vi "ReserveDbServer.vi"(0 "DashboardServer in":refnum<class "Dashboard Server.lvclass">, 5 "error in (no error)":errorcluster) -> (14 "DashboardServer out":refnum<class "Dashboard Server.lvclass">, 19 "error out":errorcluster)   [LabVIEW 2019, in "Dashboard Server.lvclass"]
uses:
  Dashboard Server.lvclass
  Dashboard Server.lvclass/Dashboard Server.ctl
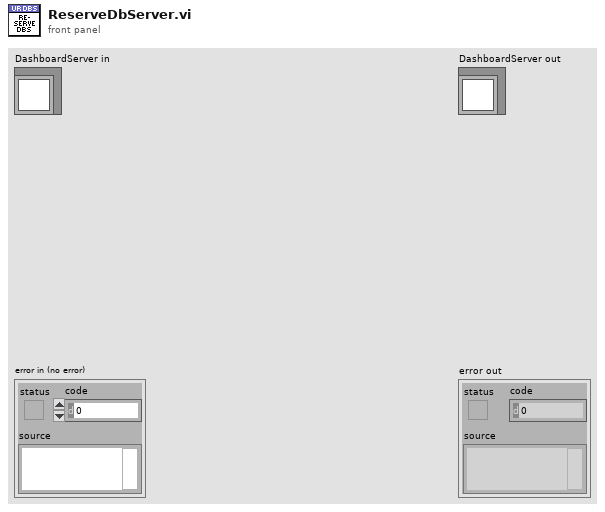
[diagram p1: front panel]
types:
  T1 = typedef "Semaphore RefNum" = refnum<k1>
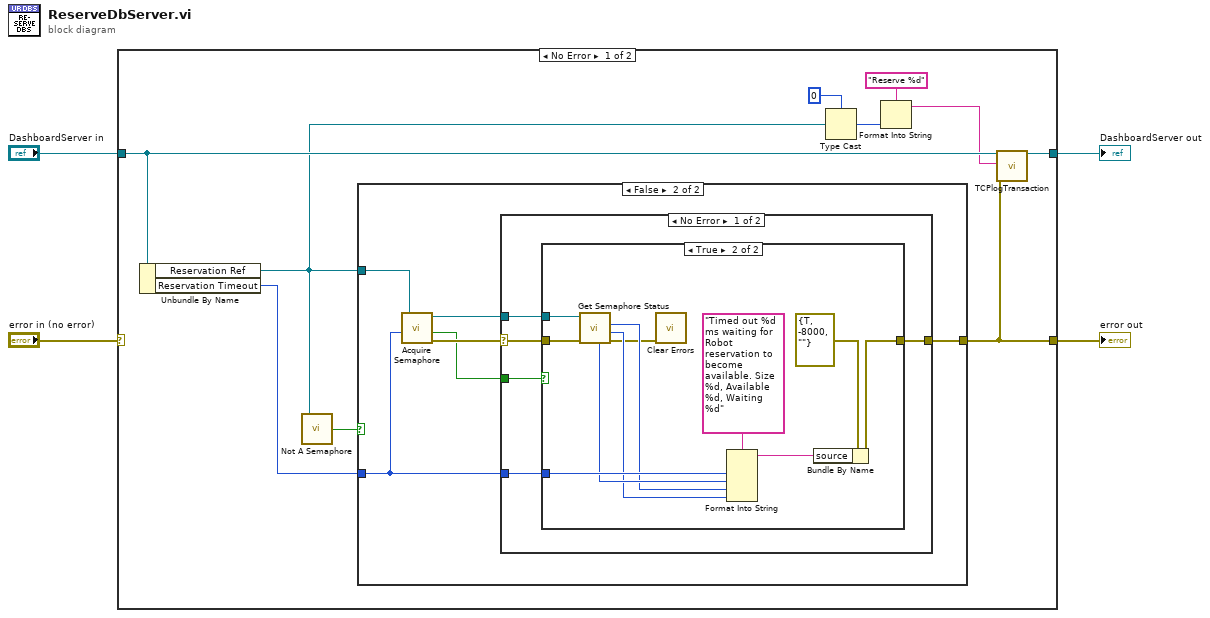
[diagram p0: block diagram]
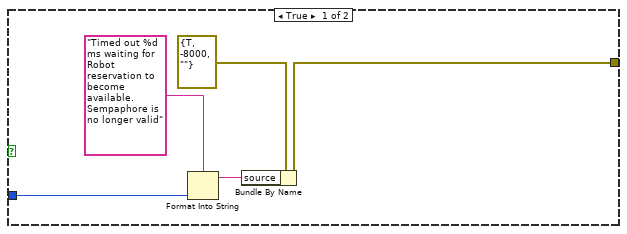
[diagram p2: hidden frame]
diagram:
  n1 = case shown="No Error" "error in (no error)" {
    selector: "error in (no error)" -> [_ w45]
    tunnel: [w8 w45] -> w3
    tunnel: [w13 w44] -> w1
    tunnel: "DashboardServer in" -> [w14 w44]
    frame No Error {
      n2 = Unbundle By Name(w14) -> ("Reservation Ref"=w6:T1, "Reservation Timeout"=w9:i32)
      n3 = call <vilib>:"Not A Semaphore.vi"("semaphore"=w6) -> ("not a semaphore"=w5:bool)
      n4 = case shown="False" w5 {
        tunnel: w9 -> [w19 w22]
        tunnel: [w18 w21] -> w8
        tunnel: w6 -> [_ w20]
        frame True {
          n5 = Format Into String(format string="Timed out %d ms waiting for Robot reservation to become available. Sempaphore is no longer valid" ("source"), w19) -> (resulting string=w17:string)  [unwired: 2 in, 1 out]
          n6 = Bundle By Name(cluster=errorcluster {"status"=TRUE, "code"=-8000, "source"=""} ("error constant"), "source"=w17) -> (w18:errorcluster)
        }
        frame False {
          n7 = call <vilib>:"Acquire Semaphore.vi"("ms timeout (-1)"=w22, "semaphore"=w20) -> ("error out"=w25:errorcluster, "timed out"=w24:bool, "semaphore out"=w23:T1)  [unwired: 3 in]
          n8 = case shown="No Error" w25 {
            selector: w25 -> [w28 w43]
            tunnel: w24 -> [w30 _]
            tunnel: w23 -> [w29 _]
            tunnel: [w27 w43] -> w21
            tunnel: w22 -> [w26 _]
            frame No Error {
              n9 = case shown="True" w30 {
                tunnel: w29 -> [_ w42]
                tunnel: w28 -> [w31 w32]
                tunnel: [w31 w40] -> w27
                tunnel: w26 -> [_ w41]
                frame False {
                }
                frame True {
                  n10 = call <vilib>:"Get Semaphore Status.vi"("error in (no error)"=w32, "semaphore"=w42) -> ("error out"=w33:errorcluster, "# waiting"=w35:i32, "# available"=w34:i32, "size"=w36:i32)  [unwired: 4 in, 2 out]
                  n11 = call <vilib>:"Clear Errors.vi"("error in (no error)"=w33) -> ()  [unwired: 5 in, 2 out]
                  n12 = Format Into String(format string="Timed out %d ms waiting for Robot reservation to become available. Size %d, Available %d, Waiting %d" ("source"), w41, w36, w34, w35) -> (resulting string=w39:string)  [unwired: 2 in, 1 out]
                  n13 = Bundle By Name(cluster=errorcluster {"status"=TRUE, "code"=-8000, "source"=""} ("error constant"), "source"=w39) -> (w40:errorcluster)
                }
              }
            }
            frame Error {
            }
          }
        }
      }
      n14 = Type Cast(type=0, x=w6) -> (*(type *) &x=w12:i32)
      n15 = Format Into String(format string="Reserve %d", w12) -> (resulting string=w10:string)  [unwired: 2 in, 1 out]
      n16 = call "TCPlogTransaction.vi"("Dashboard Server in"=w14, "Transaction"=w10, "error in (no error)"=w8) -> ("Dashboard Server out"=w13:refnum<class "Dashboard Server.lvclass">)  [unwired: 16 in]
    }
    frame Error {
    }
  }
  "error out" <- w3
  "DashboardServer out" <- w1
